vi "rspvtd_Go to MHL Case.vi"(8 "error in":errorcluster, 11 "Data in":variant) -> (0 "error out":errorcluster, 3 "Data out":T1)   [LabVIEW 2017, in "Message Log.lvclass"]
doc: "This VI converts variant data contained in the associated <b>Public API Response</b> message to its correct data type.\n---"
uses:
  Message Log.lvclass
  rsp_Go to MHL Case.ctl
  Common VIs/Message Log ID.ctl
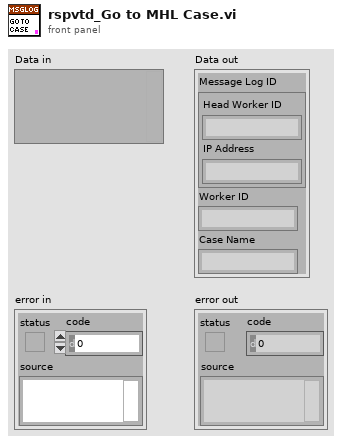
[diagram p1: front panel]
types:
  T1 = typedef "Message Log.lvclass/rsp_Go to MHL Case.ctl" = cluster{"Message Log ID":T2, "Worker ID":string, "Case Name":string}
  T2 = typedef "Message Log ID.ctl" = cluster{"Head Worker ID":string, "IP Address":string}
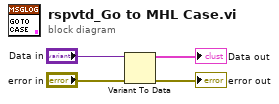
[diagram p0: block diagram]
diagram:
  n1 = Variant To Data(error in="error in", Variant="Data in") -> (data=→"Data out":T1, error out=→"error out":errorcluster)  [unwired: 1 in]
